vi "_LibDef.vi"() -> (3 "LIBNAME":string)   [LabVIEW 2017, in "StopSignal.lvlib"]
uses:
  StopSignal.lvlib
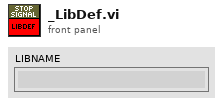
[diagram p1: front panel]
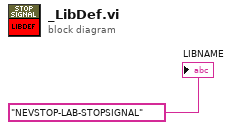
[diagram p0: block diagram]
diagram:
  "LIBNAME" <- "NEVSTOP-LAB-STOPSIGNAL" ("LIBNAME")
